vi "R3_Calibrate PR pH.vi"() -> ()   [LabVIEW 2016]
uses:
  R3_Reactor Status.ctl
  <vilib>/Analysis/NI_AALPro.lvlib
panel:
  out "Intercept":dbl
  out "Slope":dbl
  in  "Buffer Solution pH":dbl
  out "XY Graph":cluster{"Y":dbl[], "Y":dbl[]}[](graph)
  in  "Begin Calibration":bool
  in  "Number of Calibration Points":i32=3
  out "pH Amperage":dbl
  in  "Acquire":bool
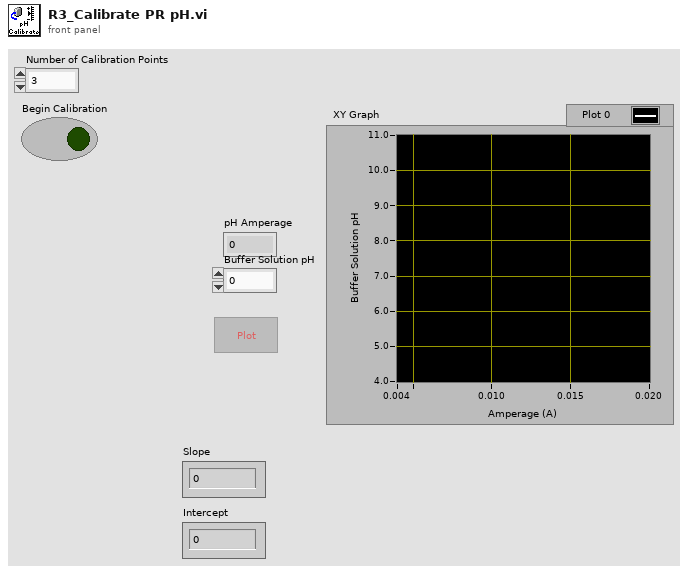
[diagram p1: front panel]
types:
  T1 = enum8{"Enabled", "Disabled", "Disabled and Grayed Out"}
  T2 = typedef "R3_Reactor Status.ctl" = cluster{"AR  Influent":bool, "AR Effluent":bool, "PR Acid":bool, "PR Base":bool, "PR Feed":bool, "PR Aeration":bool, "PR Decant":bool, "pH 1":dbl, "DO (mg/L)":dbl, "pH 1 Amp (A)":dbl, "DO Amp (A)":dbl, "PR Anoxic Feed":bool, "PR Stirrer":bool, "Reactor Status":dbl, "AR Acid":bool, "AR Base":bool, "pH 2":dbl, "pH 2 Amp (A)":dbl, "AR Stirrer":bool, "Recycle 1":bool, "Recycle 2":bool, "Combined Feed":bool}
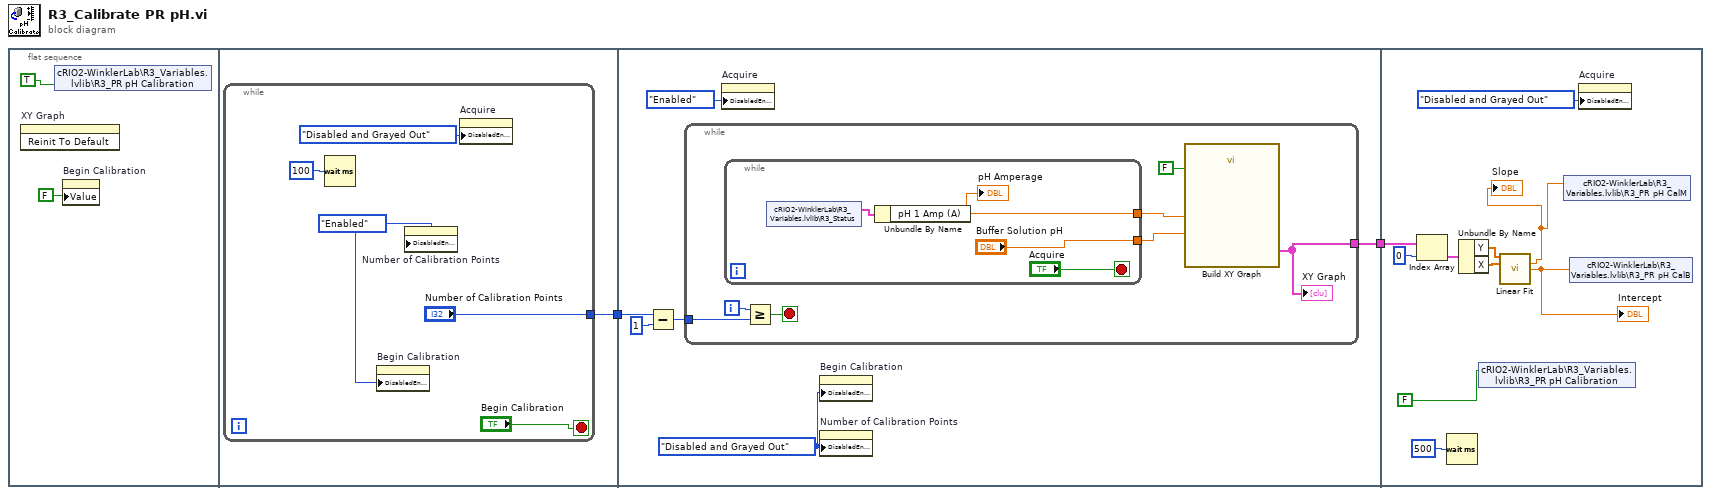
[diagram p0: block diagram]
diagram:
  n1 = flat-sequence {
    tunnel: [w5] -> w2
    tunnel: w2 -> [w13]
    tunnel: [w14] -> w1
    tunnel: w1 -> [w36]
    frame #0 {
      n2 = invoke on="XY Graph" class="XYGraph (strict)" method="Reinit To Default"() -> ()  [unwired: 3 in, 3 out]
      n3 = shared-variable "cRIO2-WinklerLab\\R3_Variables.lvlib\\R3_PR pH Calibration"(TRUE ("pH Calibration")) -> ()  [unwired: 1 in, 1 out]
      n4 = property on="Begin Calibration" class="Bool (strict)"("Value"=FALSE ("Begin Calibration")) -> ()  [unwired: 2 in, 2 out]
    }
    frame #1 {
      n5 = while {
        tunnel: ["Number of Calibration Points"] -> w5
        stop <- "Begin Calibration" stop-if-true
        w6 = T1."Enabled" ("Disabled")
        n6 = Wait (ms)(milliseconds to wait=u32 100) -> ()  [unwired: 1 out]
        n7 = property on="Begin Calibration" class="Bool (strict)"("DisabledEnum"=w6) -> ()  [unwired: 2 in, 2 out]
        n8 = property on="Number of Calibration Points" class="DigNum (strict)"("DisabledEnum"=w6) -> ()  [unwired: 2 in, 2 out]
        n9 = property on="Acquire" class="Bool"("DisabledEnum"=T1."Disabled and Grayed Out" ("Disabled")) -> ()  [unwired: 2 in, 2 out]
      }
    }
    frame #2 {
      w16 = T1."Disabled and Grayed Out" ("Disabled")
      n10 = Subtract(x=w13, y=1) -> (x-y=w11:i32)
      n11 = while {
        tunnel: w11 -> [w19]
        tunnel: [w20] -> w14
        i -> [w22]
        stop <- w23 stop-if-true
        n12 = while {
          tunnel: [w26] -> w17
          tunnel: ["Buffer Solution pH"] -> w18
          stop <- "Acquire" stop-if-true
          n13 = shared-variable "cRIO2-WinklerLab\\R3_Variables.lvlib\\R3_Status"() -> (w24:T2)  [unwired: 1 in, 1 out]
          n14 = Unbundle By Name(w24) -> ("pH 1 Amp (A)"=w26:dbl)
          "pH Amperage" <- w26
        }
        n15 = Greater Or Equal?(x=w22, y=w19) -> (x >= y?=w23:bool)
        n16 = call "Build XY Graph"("Reset"=FALSE, "Y Input"=w18, "X Input"=w17) -> ("XY Graph"=w20:cluster{"X":dbl[], "Y":dbl[]}[])  [unwired: 7 in, 1 out]
        "XY Graph" <- w20
      }
      n17 = property on="Acquire" class="Bool"("DisabledEnum"=T1."Enabled" ("Disabled")) -> ()  [unwired: 2 in, 2 out]
      n18 = property on="Begin Calibration" class="Bool (strict)"("DisabledEnum"=w16) -> ()  [unwired: 2 in, 2 out]
      n19 = property on="Number of Calibration Points" class="DigNum (strict)"("DisabledEnum"=w16) -> ()  [unwired: 2 in, 2 out]
    }
    frame #3 {
      n20 = Index Array(array=w36, index=0) -> (element=w34:cluster{"X":dbl[], "Y":dbl[]})
      n21 = Wait (ms)(milliseconds to wait=u32 500) -> ()  [unwired: 1 out]
      n22 = Unbundle By Name(w34) -> ("Y"=w33:dbl[], "X"=w32:dbl[])
      n23 = shared-variable "cRIO2-WinklerLab\\R3_Variables.lvlib\\R3_PR pH Calibration"(FALSE ("pH Calibration")) -> ()  [unwired: 1 in, 1 out]
      n24 = call <vilib>:"Linear Fit.vi"("Y"=w33, "X"=w32) -> ("slope"=w28:dbl, "intercept"=w29:dbl)  [unwired: 9 in, 3 out]
      "Slope" <- w28
      "Intercept" <- w29
      n25 = shared-variable "cRIO2-WinklerLab\\R3_Variables.lvlib\\R3_PR pH CalM"(w28) -> ()  [unwired: 1 in, 1 out]
      n26 = shared-variable "cRIO2-WinklerLab\\R3_Variables.lvlib\\R3_PR pH CalB"(w29) -> ()  [unwired: 1 in, 1 out]
      n27 = property on="Acquire" class="Bool"("DisabledEnum"=T1."Disabled and Grayed Out" ("Disabled")) -> ()  [unwired: 2 in, 2 out]
    }
  }
